vi "Constructor.vi"(8 "error in (no error)":errorcluster, 11 "Mass Flow Controller in":refnum<class "Mass Flow Controller.lvclass">) -> (0 "error out":errorcluster, 2 "Init":bool, 3 "Mass Flow Controller out":refnum<class "Mass Flow Controller.lvclass">)   [LabVIEW 2011, in "Mass Flow Controller.lvclass"]
uses:
  Mass Flow Controller.lvclass
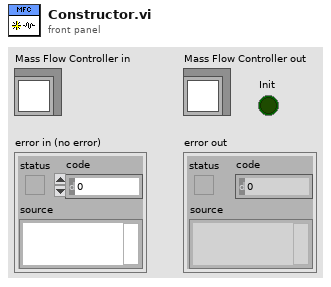
[diagram p1: front panel]
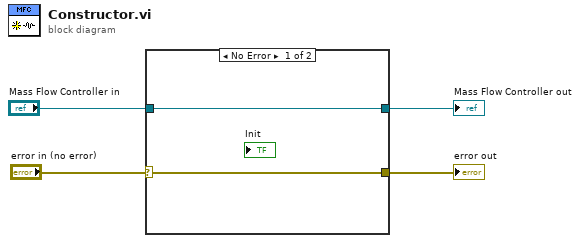
[diagram p0: block diagram]
diagram:
  n1 = case shown="No Error" "error in (no error)" {
    selector: "error in (no error)" -> [w5 w8]
    tunnel: [w5 w8] -> w3
    tunnel: [w6 w7] -> w1
    tunnel: "Mass Flow Controller in" -> [w6 w7]
    frame No Error {
    }
    frame Error {
    }
  }
  "error out" <- w3
  "Mass Flow Controller out" <- w1
